vi "Plot Label StdFormat.vi"(1 "Time Type":string, 2 "Format String":string, 3 "Type (false = numeric)":bool) -> (0 "Custom":i32)   [LabVIEW 2020, in "3D Plot.lvclass"]
uses:
  <vilib>/Math Plots/3D Math Plots/3D Plot/3D Plot/3D Plot.lvclass
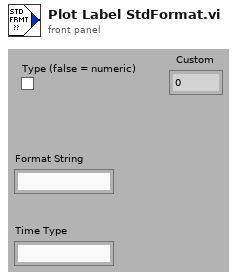
[diagram p1: front panel]
types:
  T1 = cluster{"Code Char":string, "Precision":i32, "MinWidth":u16, "EmbeddedString":string, "Modifiers":string}
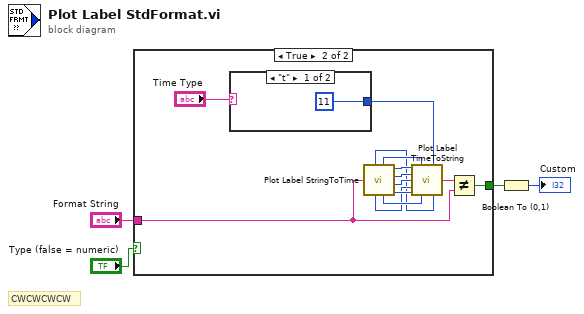
[diagram p0: block diagram]
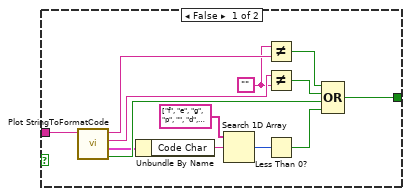
[diagram p2: hidden frame]
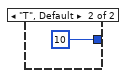
[diagram p3: hidden frame]
diagram:
  # "CWCWCWCW"
  n1 = case shown="True" "Type (false = numeric)" {
    tunnel: "Format String" -> [w17 w21]
    tunnel: [w10 w20] -> w2
    frame False {
      w14 = ""
      n2 = call <vilib>:"Plot StringToFormatCode.vi"("Start String"=w17) -> ("Error"=w11:bool, "FormatCode"=w9:T1, "Delim"=w15:string, "Remaining String"=w16:string)  [unwired: 7 out]
      n3 = Unbundle By Name(w9) -> ("Code Char"=w8:string)
      n4 = Search 1D Array(1D array=string[] ["f", "e", "g", "p", "", "d", "x", "o", "b"] ("formats"), element=w8) -> (index of element=w7:i32)  [unwired: 1 out]
      n5 = Not Equal?(x=w14, y=w16) -> (x != y?=w13:bool)
      n6 = Not Equal?(x=w15, y=w14) -> (x != y?=w12:bool)
      n7 = Less Than 0?(x=w7) -> (x < 0?=w6:bool)
      n8 = Compound Arithmetic op=OR(w13, w12, w11, w6) -> (w10:bool)
    }
    frame True {
      n9 = case shown="\"t\"" "Time Type" {
        tunnel: [11 10] -> w23
        frame "t" {
        }
        frame "T", Default {
        }
      }
      n10 = call <vilib>:"Plot Label StringToTime.vi"("Time & Date Format String"=w21) -> ("UTC"=w18:i16, "MDY"=w19:i16, "Time Format"=w25:i16, "AM/PM"=w30:i16, "included seconds"=w29:i16, "Date Format"=w26:i16, "seconds precision"=w28:i16, "Year Format"=w27:i16)  [unwired: 2 out]
      n11 = call <vilib>:"Plot Label TimeToString.vi"("AM/PM"=w30, "Time Format"=w25, "Type (10 = Absolute)"=w23, "included seconds"=w29, "seconds precision"=w28, "m-d-y sequence"=w19, "year format"=w27, "Date Format"=w26, "UTC"=w18) -> ("Format String"=w22:string)  [unwired: 2 in, 4 out]
      n12 = Not Equal?(x=w22, y=w21) -> (x != y?=w20:bool)
    }
  }
  n13 = Boolean To (0,1)(Boolean=w2) -> (0, 1=→"Custom":i16)
